vi "Control de frecuencia 4t 2.0.vi"() -> ()   [LabVIEW 2010]
doc: "This VI demonstrates how to output continuous sound using SO Set Num Buffers."
uses:
  <vilib>/sound/lvsound.llb/Sound Format.ctl
  <vilib>/measure/NI_MABase.lvlib
  user32.dll
panel:
  in  "Retraso foto":i32=80
  out "Foto":bool=TRUE
  in  "Punto de \noperación":bool
  in  "Amplitud":dbl(knob)=10000.0 scale=0.0..10000.0 scale format="%#_6p"
  out "Máximo":bool=TRUE
  in  "Conmutador":bool
  in  "Tasa de incremento 2":dbl format="%#_6f"
  in  "t max":u32=130
  out "Estable":bool=TRUE
  out "tiempo":u32
  in  "Encender gráfico":bool
  out "Waveform Graph":waveform(dbl)(graph)
  in  "Número de buffers":i32(slide)=5 scale=0.0..100.0
  in  "FIN":bool
  in  "Número de\nPlanos":u8=5
  in  "Frecuencia":sgl(slide) scale=0.0..5000.0
  in  "Incrementa\n frecuencia":bool
  out "Plano":u8
  out "error out":errorcluster
  # "90º"
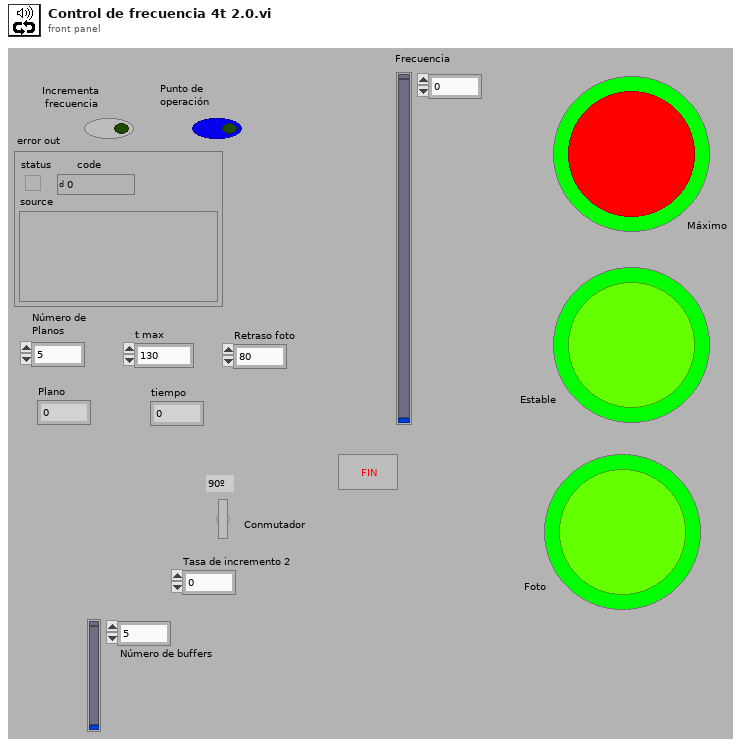
[diagram p1: front panel]
types:
  T1 = typedef "Sound Format.ctl" = cluster{"sound quality":enum16{"mono", "stereo"}, "rate":enum16{"11025", "22050", "44100", "8000"}, "bits per sample":enum16{"8 bit", "16 bit"}}
  T2 = cluster{"Extended Virtual Key List":u16, "dwFlags":u32}[]
  T3 = cluster{"Extended Virtual Key List":u16, "dwFlags":u32}
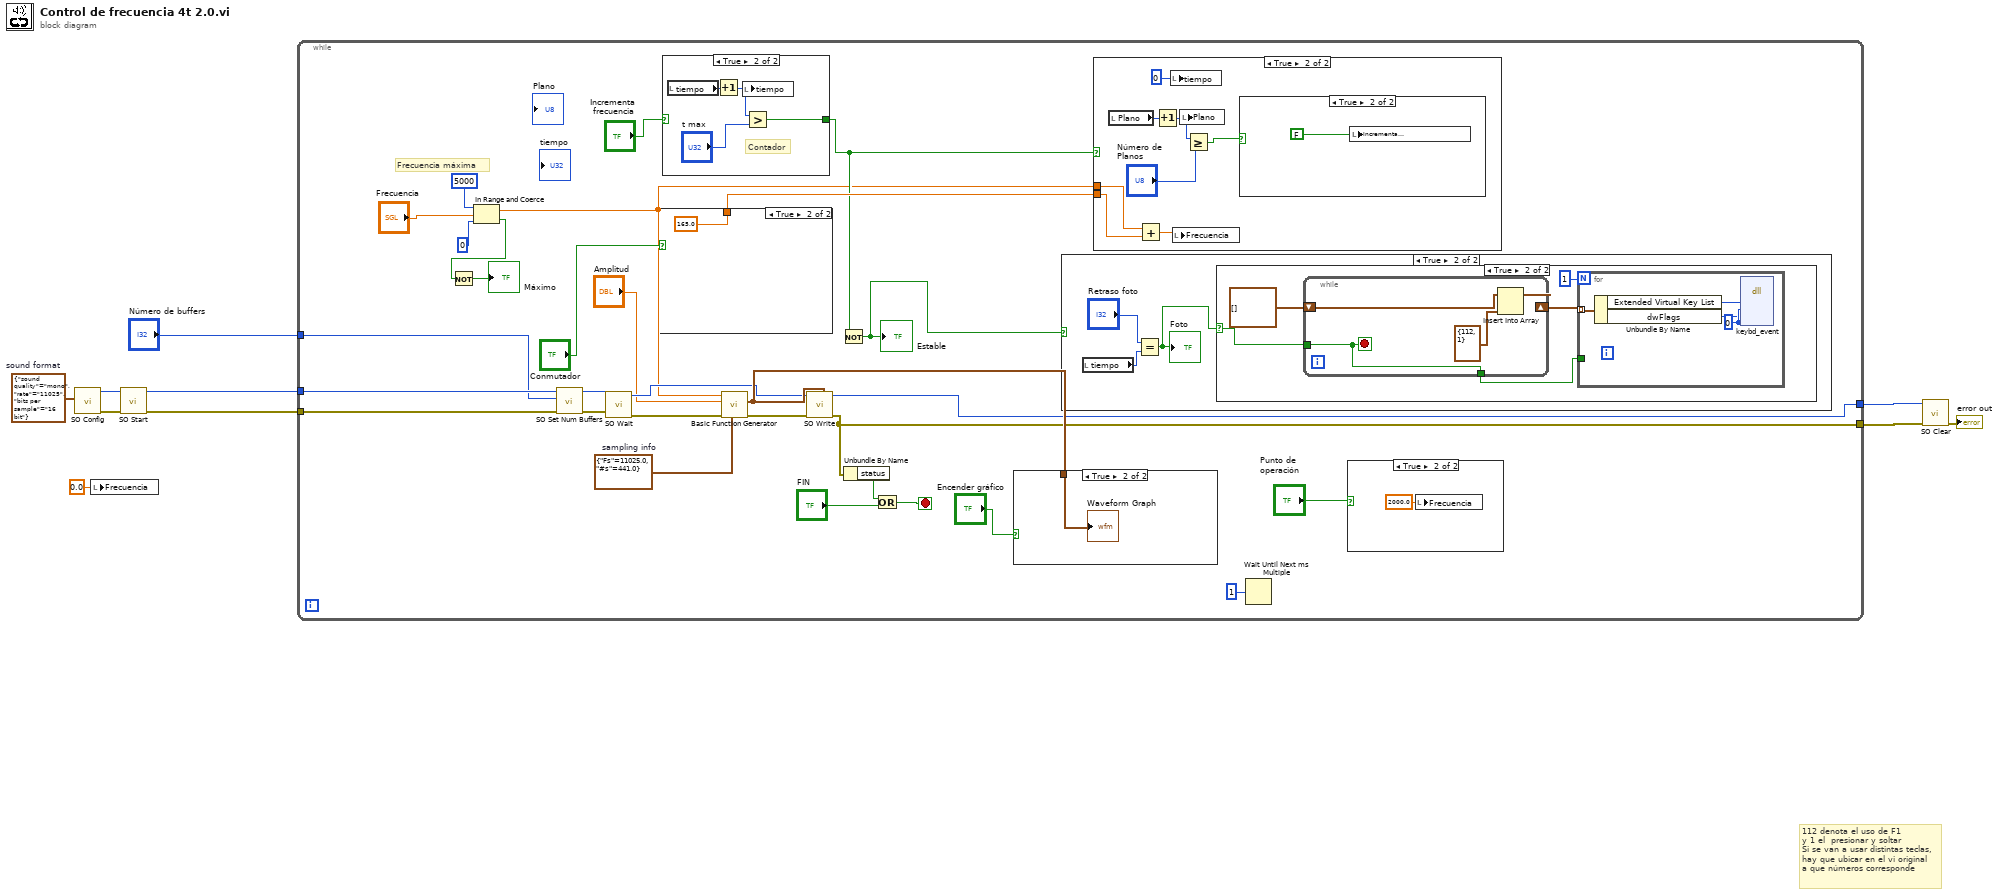
[diagram p0: block diagram]
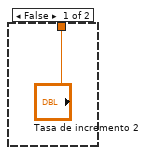
[diagram p5: hidden frame]
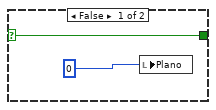
[diagram p6: hidden frame]
diagram:
  w10 = T1 {"sound quality"=enum."mono", "rate"=enum."11025", "bits per sample"=enum."16 bit"}  # sound format
  # "112 denota el uso de F1\ny 1 el  presionar y soltar\nSi se van a usar distintas teclas,\nhay que ubicar en el vi original \na que números corresponde"
  n1 = call <vilib>:"SO Config.vi"("sound format"=w10) -> ("error out"=w8:errorcluster, "task ID out"=w9:u32)  [unwired: 9 in]
  n2 = local write "Frecuencia"(0.0 ("Frecuencia")) -> ()
  n3 = call <vilib>:"SO Start.vi"("error in (no error)"=w8, "task ID in"=w9) -> ("error out"=w4:errorcluster, "task ID out"=w3:u32)  [unwired: 8 in]
  n4 = while {
    tunnel: [w33] -> w6
    tunnel: [w32] -> w5
    tunnel: w4 -> [w27]
    tunnel: w3 -> [w26]
    tunnel: "Número de buffers" -> [w25]
    stop <- w34 stop-if-true
    w37 = cluster{"Fs":dbl, "#s":dbl} {"Fs"=11025.0, "#s"=441.0}  # sampling info
    # "Frecuencia máxima"
    n5 = In Range and Coerce(upper limit=5000, x="Frecuencia", lower limit=0) -> (coerced(x)=w20:sgl, In Range?=w16:bool)
    n6 = Not(x=w16) -> (.not. x?=→"Máximo":bool)
    n7 = call <vilib>:"SO Set Num Buffers.vi"("error in (no error)"=w27, "number of buffers"=w25, "task ID in"=w26) -> ("error out"=w31:errorcluster, "task ID out"=w30:u32)  [unwired: 7 in]
    n8 = call <vilib>:"SO Wait.vi"("error in (no error)"=w31, "task ID in"=w30) -> ("error out"=w28:errorcluster, "task ID out"=w29:u32)  [unwired: 8 in]
    n9 = case shown="True" "Conmutador" {
      tunnel: ["Tasa de incremento 2" 165.0 ("Tasa de incremento 1")] -> w40
      frame False {
      }
      frame True {
      }
    }
    n10 = case shown="True" "Incrementa\n frecuencia" {
      selector: "Incrementa\n frecuencia" -> [w61 _]
      tunnel: [w61 w62] -> w22
      frame False {
        n11 = local write "Plano"(u8 0 ("Tic")) -> ()
      }
      frame True {
        # "Contador"
        n12 = local read "tiempo"() -> (w64:u32)
        n13 = Increment(x=w64) -> (x+1=w65:u32)
        n14 = local write "tiempo"(w65) -> ()
        n15 = Greater?(x=w65, y="t max") -> (0:w62:bool)
      }
    }
    n16 = call <vilib>:"Basic Function Generator.vi"("sampling info"=w37, "error in (no error)"=w28, "amplitude"="Amplitud", "frequency"=w20) -> ("error out"=w38:errorcluster, "signal out"=w35:waveform(dbl))  [unwired: 5 in, 1 out]
    n17 = call <vilib>:"SO Write.vi"("mono 16-bit"=w35, "error in (no error)"=w38, "task ID in"=w29) -> ("error out"=w32:errorcluster, "task ID out"=w33:u32)  [unwired: 7 in]
    n18 = Not(x=w22) -> (.not. x?=w11:bool)
    "Estable" <- w11
    n19 = Unbundle By Name(w32) -> ("status"=w39:bool)
    n20 = Or(x=w39, y="FIN") -> (x .or. y?=w34:bool)
    n21 = case shown="True" "Encender gráfico" {
      tunnel: w35 -> [_ w66]
      frame False {
      }
      frame True {
        "Waveform Graph" <- w66
      }
    }
    n22 = case shown="True" w11 {
      frame False {
      }
      frame True {
        n23 = local read "tiempo"() -> (w43:u32)
        n24 = Equal?(x="Retraso foto", y=w43) -> (x = y?=w41:bool)
        "Foto" <- w41
        n25 = case shown="True" w41 {
          selector: w41 -> [_ w44]
          frame False {
          }
          frame True {
            n26 = while {
              tunnel: [w49] -> w47
              shift-right: [w51] -> w48
              shift-left: T2 [] -> [w52]
              tunnel: w44 -> [w49]
              stop <- w49 stop-if-true
              n27 = Insert Into Array(array=w52, new element=T3 {"Extended Virtual Key List"=112, "dwFlags"=1} ("new element/subarray")) -> (w51:T2)  [unwired: 1 in]
            }
            n28 = for {
              N: 1 -> [_]
              tunnel: w48 -> [w54] mode=indexing
              tunnel: w47 -> [_]
              w56 = u32 0 ("dwFlags")
              n29 = Unbundle By Name(w54) -> ("Extended Virtual Key List"=w53:u16, "dwFlags"=w55:u32)
              n30 = dll-call lib="user32.dll" fn="keybd_event"("bVk"=w53, "bScan"=w56, "dwFlags"=w55, "dwExtraInfo"=w56) -> ()  [unwired: 8 in, 2 out]
            }
          }
        }
      }
    }
    n31 = case shown="True" w22 {
      tunnel: w20 -> [_ w67]
      tunnel: w40 -> [_ w70]
      frame False {
      }
      frame True {
        n32 = local read "Plano"() -> (w74:u8)
        n33 = Add(x=w67, y=w70) -> (x+y=w69:dbl)
        n34 = Increment(x=w74) -> (x+1=w73:u8)
        n35 = local write "tiempo"(u8 0 ("Tic")) -> ()
        n36 = local write "Frecuencia"(w69) -> ()
        n37 = local write "Plano"(w73) -> ()
        n38 = Greater Or Equal?(x=w73, y="Número de\nPlanos") -> (x >= y?=w71:bool)
        n39 = case shown="True" w71 {
          frame False {
          }
          frame True {
            n40 = local write "Incrementa\n frecuencia"(FALSE ("Incrementa frecuencia 2")) -> ()
          }
        }
      }
    }
    n41 = Wait Until Next ms Multiple(millisecond multiple=u32 1) -> ()  [unwired: 1 out]
    n42 = case shown="True" "Punto de \noperación" {
      frame False {
      }
      frame True {
        n43 = local write "Frecuencia"(sgl 2000.0 ("Frecuencia")) -> ()
      }
    }
  }
  n44 = call <vilib>:"SO Clear.vi"("error in (no error)"=w5, "task ID in"=w6) -> ("error out"=→"error out":errorcluster)  [unwired: 9 in]
